vi "RamCtrl_Abs_PoseEst_Exec.vi"() -> (0 "Abs Pose Est SI":T1 {"ROTATION"."SIN" format="%13.4f"; "ROTATION"."COS" format="%13.4f"; "ROTATION"."VALUE" format="%13.4f"; "TRANSLATION"."Y" format="%14.3f"; "TRANSLATION"."X" format="%14.3f"})   [LabVIEW 2019]
uses:
  <vilib>/Rock Robotics/WPI/ThirdParty/JAS_Junk/TrajLib/TypeDef/POSE2D.ctl
  <vilib>/Rock Robotics/WPI/ThirdParty/JAS_Junk/TrajLib/TypeDef/TRANSLATION2D.ctl
  <vilib>/Rock Robotics/WPI/ThirdParty/JAS_Junk/TrajLib/TypeDef/ROTATION2D.ctl
  <vilib>/Rock Robotics/WPI/ThirdParty/JAS_Junk/TrajLib/VI/numCmd_ObtainQueue_Array.vi
  <vilib>/Rock Robotics/WPI/ThirdParty/JAS_Junk/TrajLib/Trajectory_Library.lvlib
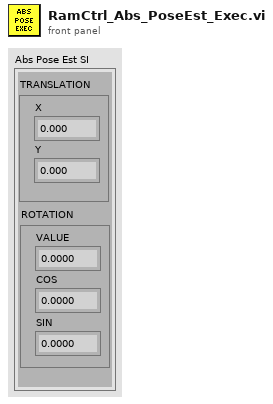
[diagram p1: front panel]
types:
  T1 = typedef "Trajectory_Library.lvlib/POSE2D.ctl" = cluster{"TRANSLATION":T2, "ROTATION":T3}
  T2 = typedef "Trajectory_Library.lvlib/TRANSLATION2D.ctl" = cluster{"X":dbl, "Y":dbl}
  T3 = typedef "Trajectory_Library.lvlib/ROTATION2D.ctl" = cluster{"VALUE":dbl, "COS":dbl, "SIN":dbl}
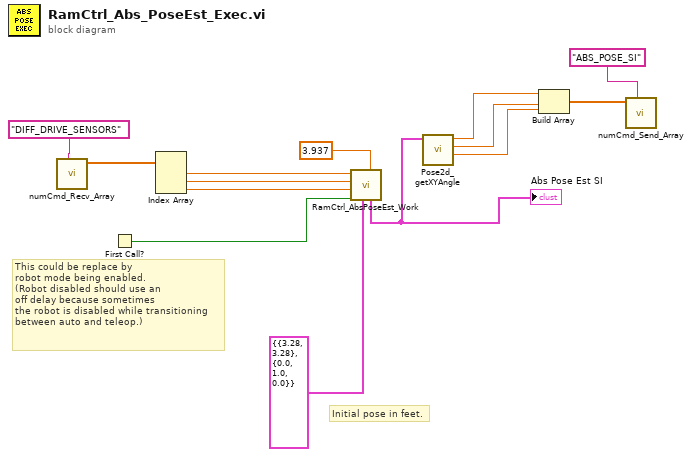
[diagram p0: block diagram]
diagram:
  # "Initial pose in feet."
  # "This could be replace by\nrobot mode being enabled.\n(Robot disabled should use an\noff delay because sometimes\nthe robot is disabled while transitioning\nbetween auto and teleop.)"
  n1 = call <vilib>:"numCmd_Recv_Array.vi"("Command Name"="DIFF_DRIVE_SENSORS") -> ("Values"=w13:dbl[])  [unwired: 8 in, 2 out]
  n2 = First Call?() -> (First Call?: T/F=w8:bool)
  n3 = Index Array(array=w13) -> (element #1=w11:dbl, element #2=w10:dbl, element #3=w9:dbl)  [unwired: 3 in]
  n4 = call "RamCtrl_AbsPoseEst_Work.vi"("Track Width FT"=3.937, "InitialPose FT"=T1 {"TRANSLATION"={"X"=3.28, "Y"=3.28}, "ROTATION"={"VALUE"=0.0, "COS"=1.0, "SIN"=0.0}}, "Init"=w8, "Gyro Continous\n (inc counterclockwise)\nDEG"=w9, "Right Distance FT"=w10, "Left Distance FT"=w11) -> ("Odometry Pose Meters"=w5:T1)  [unwired: 5 in]
  "Abs Pose Est SI" <- w5
  n5 = call <vilib>:"Pose2d_getXYAngle.vi"("in POSE"=w5) -> ("Angle"=w2:dbl, "Y"=w3:dbl, "X"=w4:dbl)  [unwired: 8 in]
  n6 = Build Array(w4, w3, w2) -> (w7:dbl[])
  n7 = call <vilib>:"numCmd_Send_Array.vi"("Command Name"="ABS_POSE_SI", "Values"=w7) -> ()  [unwired: 9 in, 1 out]
